vi "Write file descriptor.vi"(8 "error in (no error)":errorcluster, 10 "file descriptor":i32, 11 "Shared Memory in":refnum<class "Shared Memory.lvclass">) -> (0 "error out":errorcluster, 3 "Shared Memory out":refnum<class "Shared Memory.lvclass">)   [LabVIEW 2013, in "Linux RT IPC.Shared Memory.lvlib" / "Shared Memory.lvclass"]
uses:
  Shared Memory.lvclass
  Shared Memory.lvclass/Shared Memory.ctl
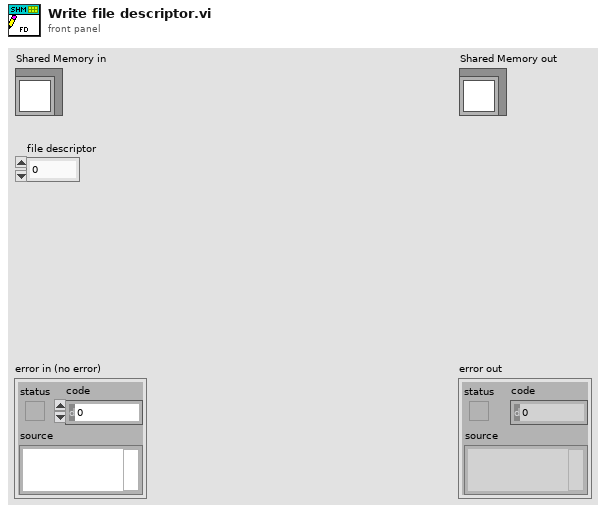
[diagram p1: front panel]
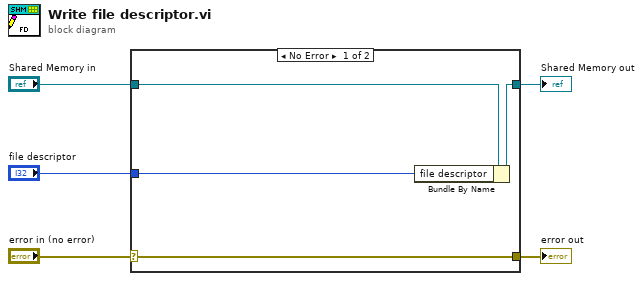
[diagram p0: block diagram]
diagram:
  n1 = case shown="No Error" "error in (no error)" {
    selector: "error in (no error)" -> [w9 w10]
    tunnel: [w9 w10] -> w4
    tunnel: [w7 w11] -> w2
    tunnel: "Shared Memory in" -> [w8 w11]
    tunnel: "file descriptor" -> [w6 _]
    frame No Error {
      n2 = Bundle By Name(cluster=w8, "file descriptor"=w6) -> (w7:refnum<class "Shared Memory.lvclass">)
    }
    frame Error {
    }
  }
  "error out" <- w4
  "Shared Memory out" <- w2
